vi "G#Object_IsExternalCreateProcessRunning.vi"(5 "error in (no error)":errorcluster) -> (15 "external create enabled?":bool, 16 "owned by external process?":bool, 17 "external create process running?":bool, 19 "error out":errorcluster)   [LabVIEW 2017, in "G#Object.lvclass"]
doc: "Checks if external create is enabled and also if the external create process is running."
uses:
  G#Object.lvclass
  <vilib>/Utility/error.llb/Error Cluster From Error Code.vi
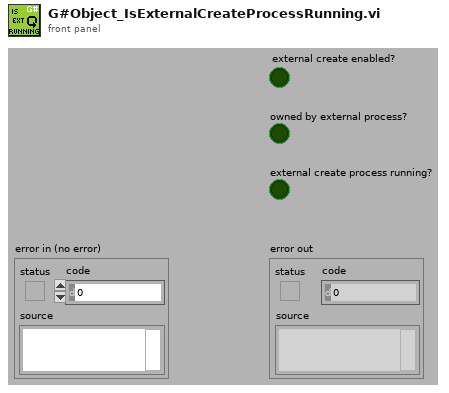
[diagram p1: front panel]
types:
  T1 = enum32{"Bad", "Idle", "Run top level", "Running"}
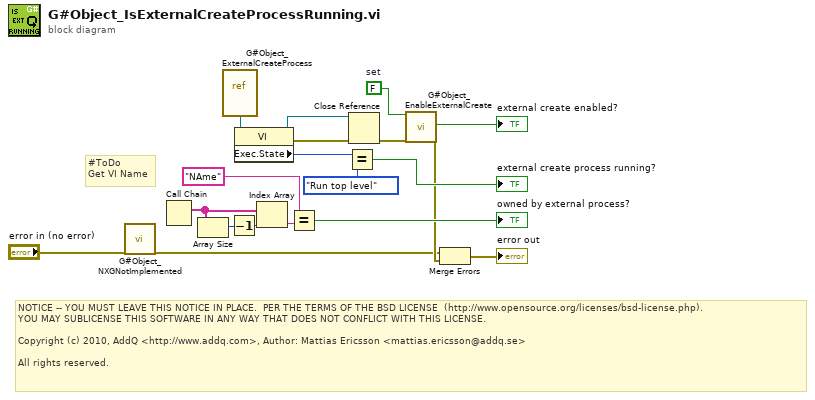
[diagram p0: block diagram]
diagram:
  w10 = FALSE  # set
  # "#ToDo\nGet VI Name"
  # "NOTICE -- YOU MUST LEAVE THIS NOTICE IN PLACE.  PER THE TERMS OF THE BSD LICENSE  (http://www.opensource.org/licenses/bsd-license.php).\nYOU MAY SUBLICENSE THIS SOFTWARE IN ANY WAY THAT DOES NOT CONFLICT WITH THIS LICENSE.\n\nCopyright (c) 2010, AddQ <http://www.addq.com>, Author: Mattias Ericsson <mattias.ericsson@addq.se>\n\nAll rights reserved."
  n1 = call "G#Object_NXGNotImplemented.vi"("error in"="error in (no error)") -> ("error out"=w2:errorcluster)  [unwired: 18 in]
  n2 = Call Chain() -> (call chain=w9:string[])
  n3 = Array Size(array=w9) -> (size(s)=w7:i32)
  n4 = vi-ref "G#Object_ExternalCreateProcess.vi"() -> (w16:refnum<vi>)
  n5 = Decrement(x=w7) -> (x-1=w6:i32)
  n6 = property class="VI"(reference=w16) -> (reference out=w14:refnum<vi>, error out=w15:errorcluster, "Exec.State"=w13:T1)  [unwired: 1 in]
  n7 = Index Array(array=w9, index=w6) -> (element=w8:string)
  n8 = Equal?(x="NAme", y=w8) -> (x = y?=→"owned by external process?":bool)
  n9 = Equal?(x=w13, y=T1."Run top level" ("Execution:State")) -> (x = y?=→"external create process running?":bool)
  n10 = Close Reference(reference=w14, error in (no error)=w15) -> (error out=w11:errorcluster)
  n11 = call "G#Object_EnableExternalCreate.vi"("set (F)"=w10, "error in (no error)"=w11) -> ("enabled"=→"external create enabled?":bool, "error out"=w5:errorcluster)  [unwired: 15 in, 1 out]
  n12 = Merge Errors(w2, w5) -> (→"error out":errorcluster)
